vi "创建新工作表.vi"(7 "新工作表名称":string, 8 "错误输入（无错误）":errorcluster, 11 "引用簇":T1) -> (0 "错误输出":errorcluster, 2 "新工作表":refnum<k7>, 3 "引用簇输出":T1, 5 "新工作表名称输出":string)   [LabVIEW 2020, in "OperateExcel.lvlib"]
uses:
  OperateExcel.lvlib
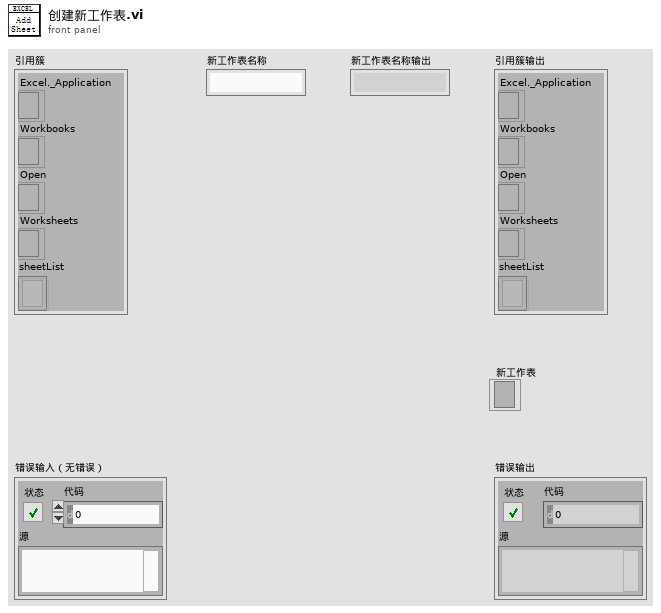
[diagram p1: front panel]
types:
  T1 = typedef "OperateExcel.lvlib/引用簇.ctl" = cluster{"Excel._Application":refnum<k7>, "Workbooks":refnum<k7>, "Open":refnum<k7>, "Worksheets":refnum<k7>, "sheetList":refnum<k7>[]}
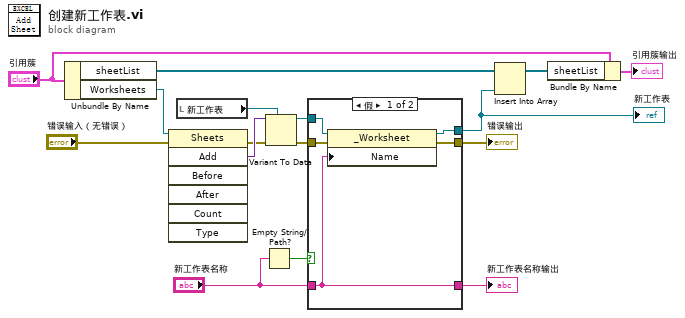
[diagram p0: block diagram]
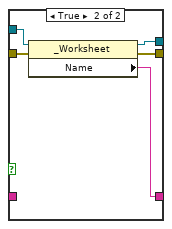
[diagram p2: hidden frame]
diagram:
  n1 = Unbundle By Name("引用簇") -> ("sheetList"=w7:refnum<k7>[], "Worksheets"=w2:refnum<k7>)
  n2 = invoke class="Sheets" method="Add"(reference=w2, error in="错误输入（无错误）") -> (error out=w14:errorcluster, "Add"=w16:variant)  [unwired: 5 in, 5 out]
  n3 = local read "新工作表"() -> (w1:refnum<k7>)
  n4 = Empty String/Path?(string/path="新工作表名称") -> (empty?=w10:bool)
  n5 = Variant To Data(error in=w14, type=w1, Variant=w16) -> (data=w15:refnum<k7>, error out=w13:errorcluster)
  n6 = case shown="假" w10 {
    tunnel: w15 -> [w21 w26]
    tunnel: "新工作表名称" -> [w17 _]
    tunnel: [w20 w24] -> w6
    tunnel: w13 -> [w19 w25]
    tunnel: [w18 w23] -> w12
    tunnel: [w17 w22] -> w8
    frame False {
      n7 = property class="_Worksheet"(reference=w21, error in=w19, "Name"=w17) -> (reference out=w20:refnum<k7>, error out=w18:errorcluster)
    }
    frame True {
      n8 = property class="_Worksheet"(reference=w26, error in=w25) -> (reference out=w24:refnum<k7>, error out=w23:errorcluster, "Name"=w22:string)
    }
  }
  "新工作表" <- w6
  "错误输出" <- w12
  "新工作表名称输出" <- w8
  n9 = Insert Into Array(array=w7, new element=w6) -> (w4:refnum<k7>[])  [unwired: 1 in]
  n10 = Bundle By Name(cluster="引用簇", "sheetList"=w4) -> (→"引用簇输出":T1)
